vi "TemplateDaemonTester.vi"() -> ()   [LabVIEW 2024]
uses:
  TemplateDaemon_class/status--cluster.ctl
  TemplateDaemon_class/states--enum.ctl
  TemplateDaemon_class/TemplateDaemon.lvclass
  <vilib>/addons/_JKI Toolkits/State Machine/_JKI_lib_State_Machine.llb/Select State(s)_err__jki_lib_state_machine.vi
panel:
  in  "loop period (ms)":i32
  in  "set period":bool
  out "current status":T1
  in  "stop daemon":bool
  in  "start daemon":bool
  in  "destroy daemon":bool
  in  "create daemon":bool
  in  "Exit":bool
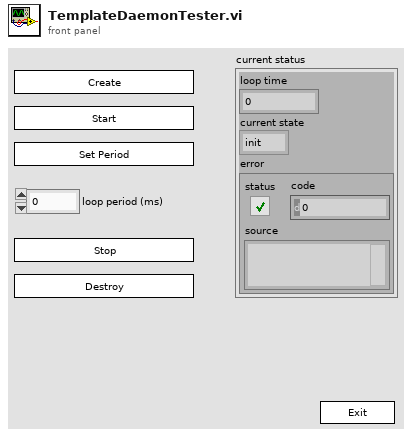
[diagram p1: front panel]
types:
  T1 = typedef "TemplateDaemon.lvclass/status--cluster.ctl" = cluster{"loop time":u32, "current state":T2, "error":errorcluster}
  T2 = typedef "TemplateDaemon.lvclass/states--enum.ctl" = enum16{"init", "default", "error handler", "exit"}
  T3 = enum32{"Invalid", "Standard", "Closed", "Hidden", "Minimized", "Maximized"}
  T4 = enum32{"invalid app kind", "Development System", "Run Time System", "Student Edition", "Embedded LabVIEW", "Evaluation", "Custom"}
  T5 = cluster{"Core":cluster{"Current VI Reference":refnum<vi>, "Close Panel on Exit?":bool}, "TemplateDaemon":refnum<class "TemplateDaemon.lvclass">, "TO":i32}
  T6 = cluster{"Current VI Reference":refnum<vi>, "Close Panel on Exit?":bool}
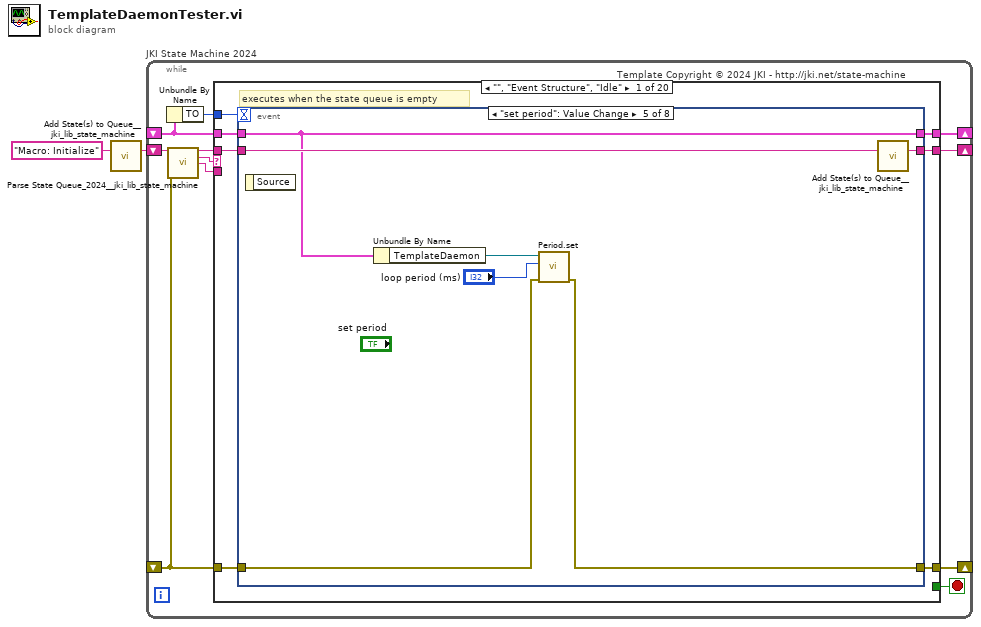
[diagram p0: block diagram]
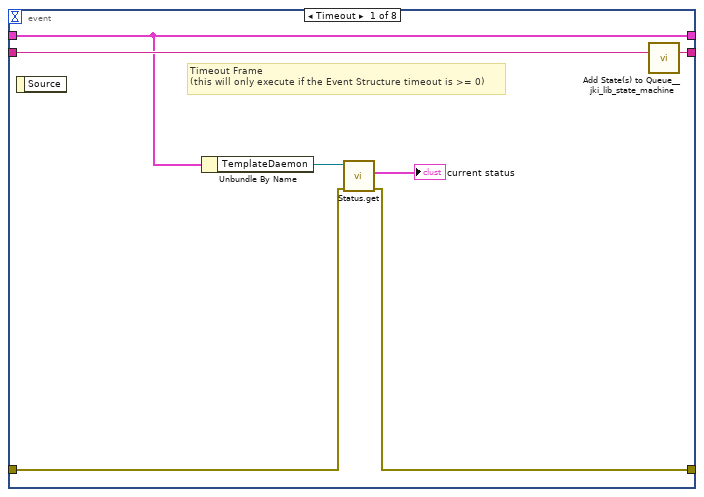
[diagram p2: hidden frame]
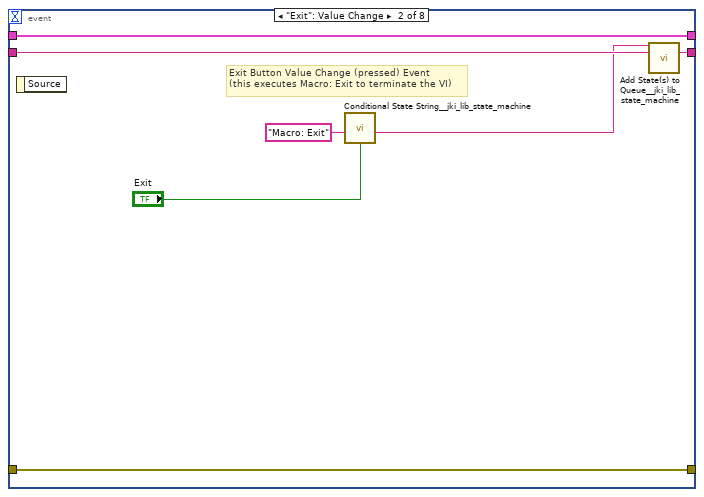
[diagram p3: hidden frame]
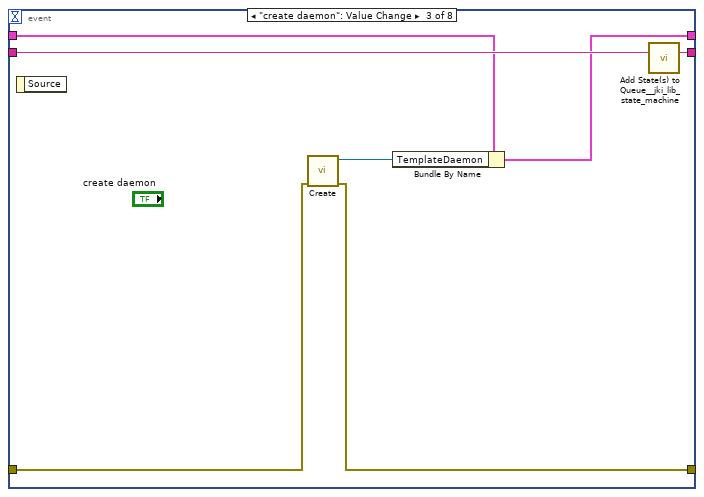
[diagram p4: hidden frame]
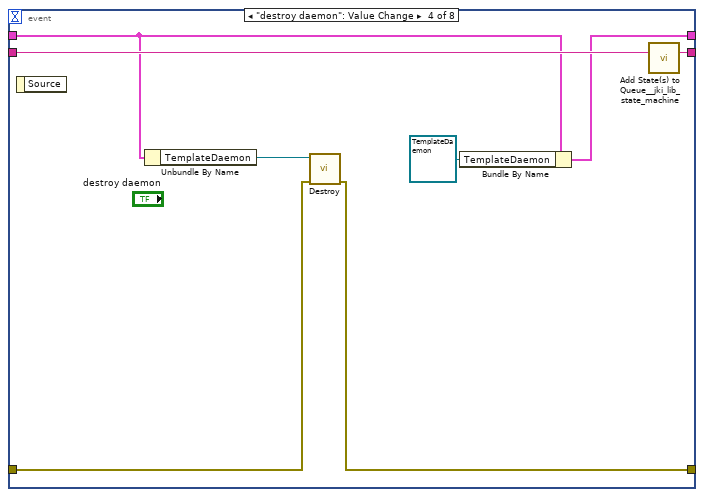
[diagram p5: hidden frame]
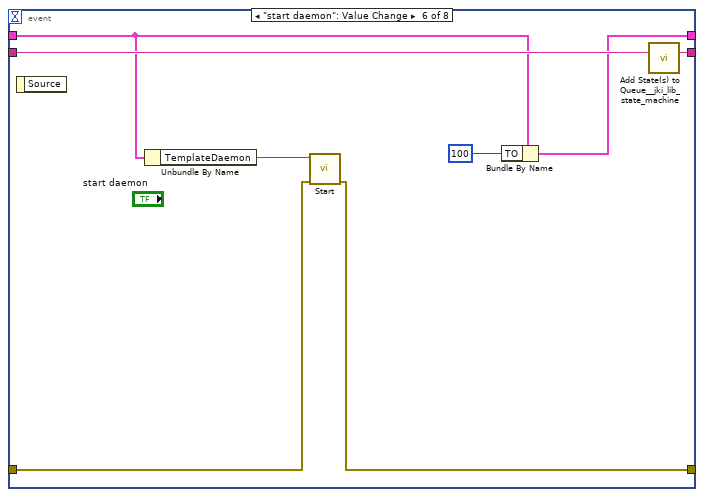
[diagram p6: hidden frame]
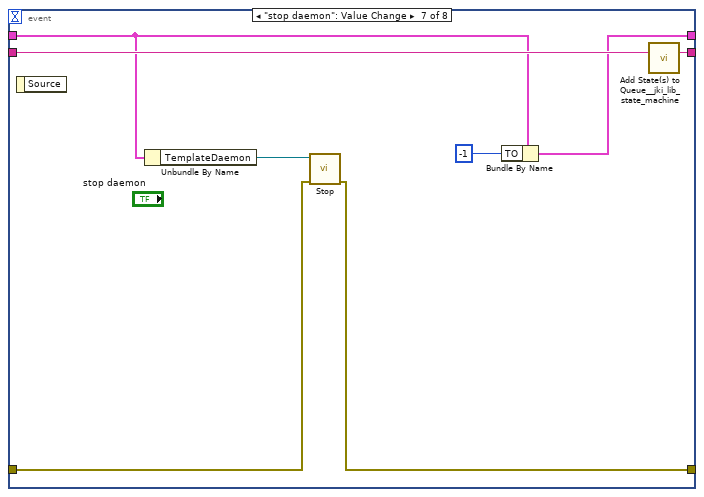
[diagram p7: hidden frame]
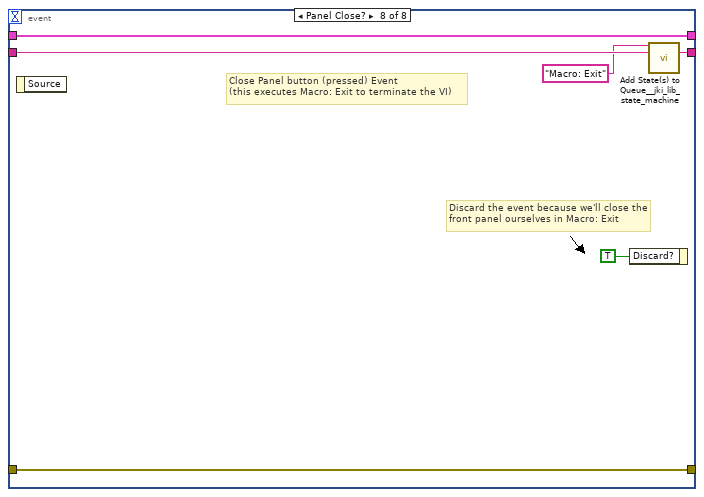
[diagram p8: hidden frame]
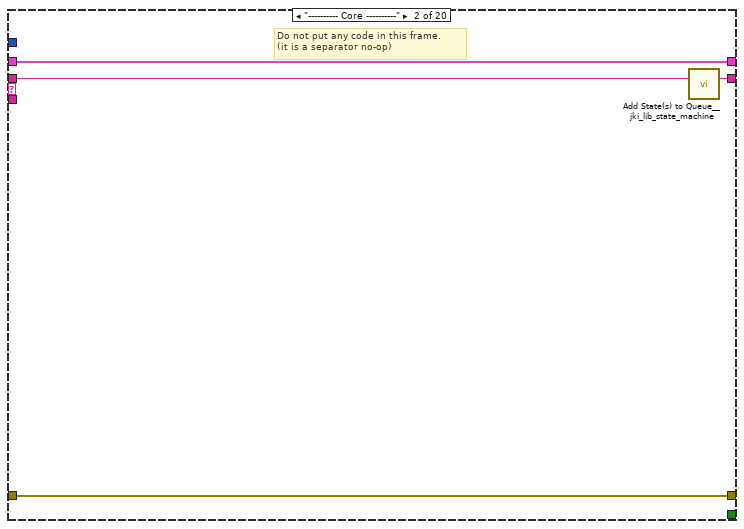
[diagram p9: hidden frame]
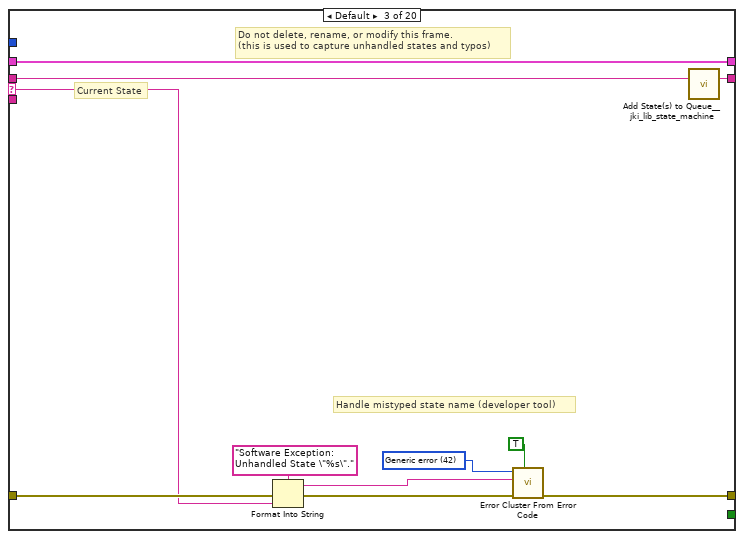
[diagram p10: hidden frame]
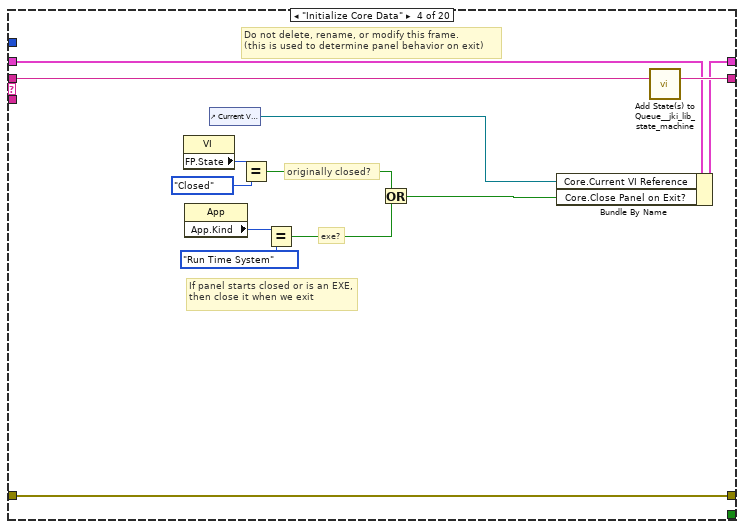
[diagram p11: hidden frame]
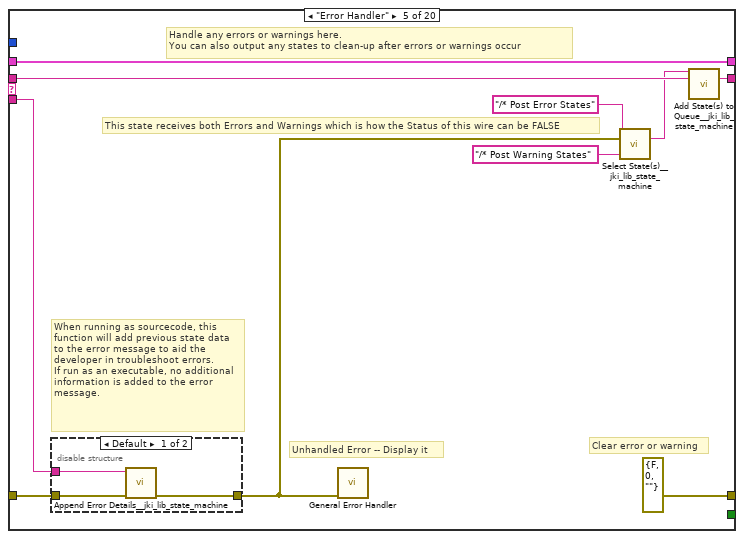
[diagram p12: hidden frame]
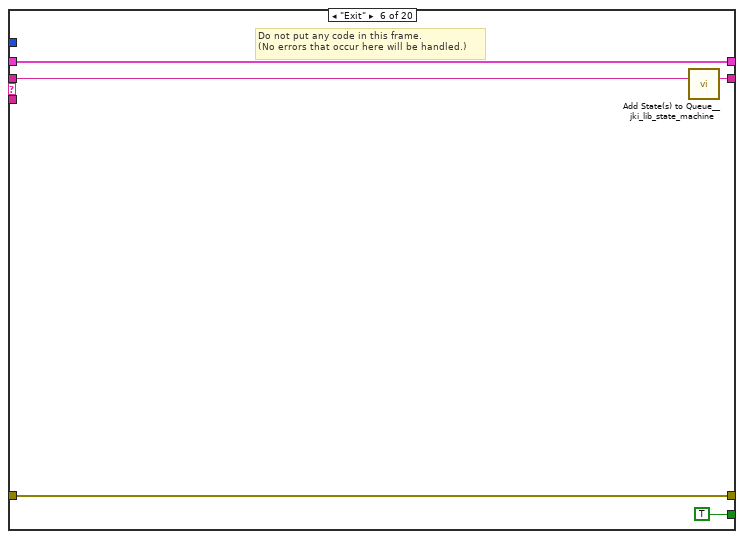
[diagram p14: hidden frame]
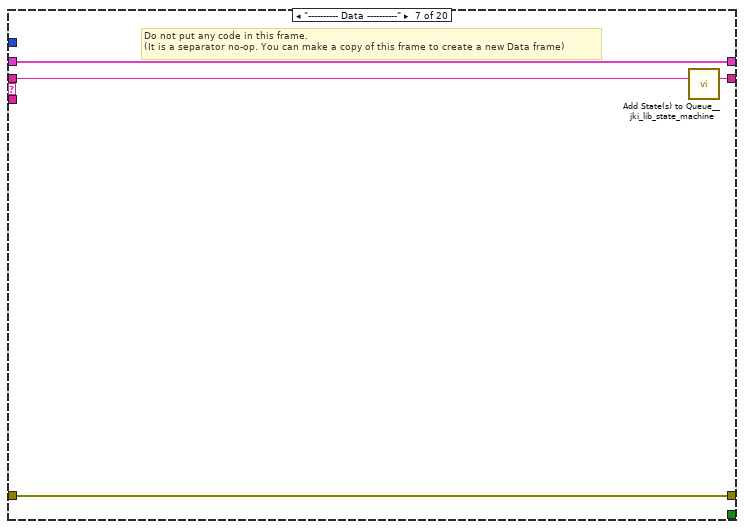
[diagram p15: hidden frame]
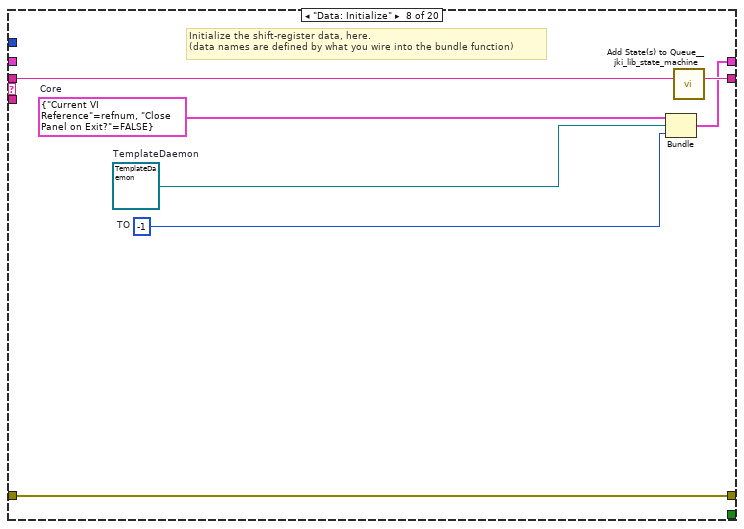
[diagram p16: hidden frame]
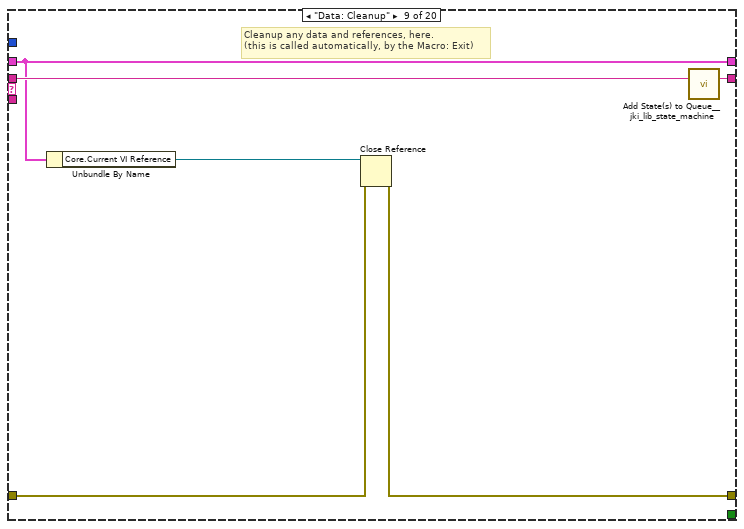
[diagram p17: hidden frame]
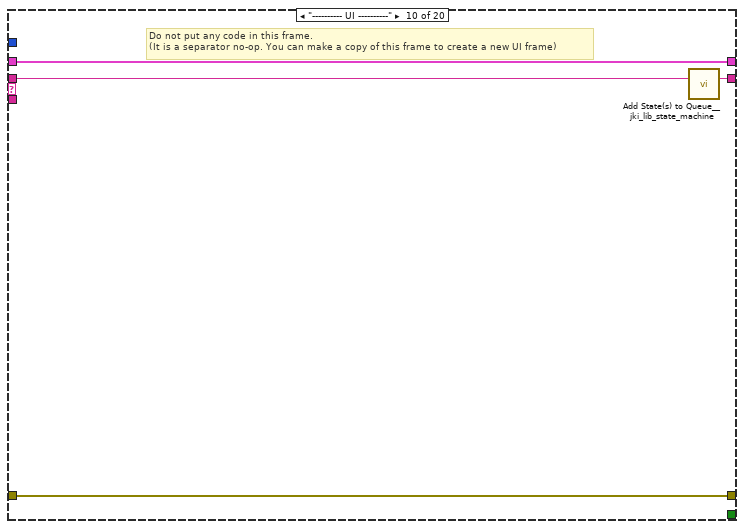
[diagram p18: hidden frame]
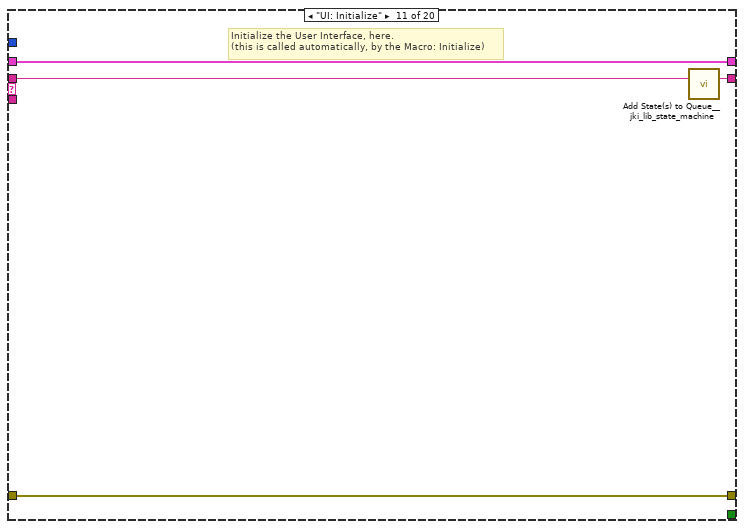
[diagram p19: hidden frame]
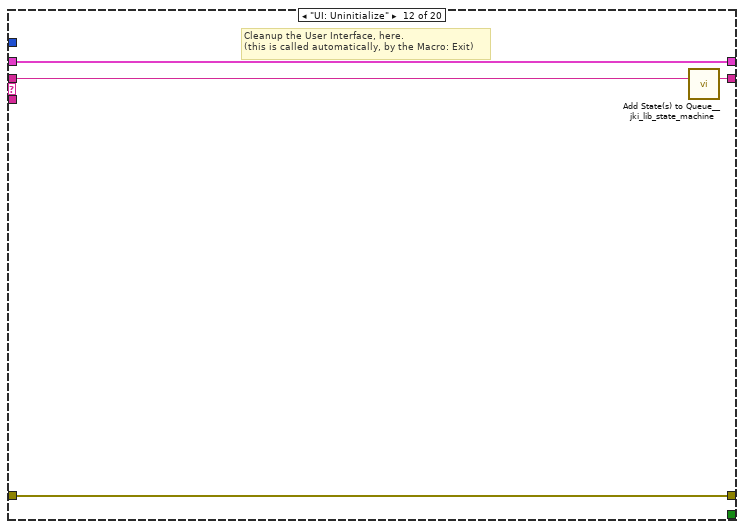
[diagram p20: hidden frame]
diagram:
  n1 = call <vilib>:"Add State(s) to Queue__jki_lib_state_machine.vi"("State(s) in (\"\")"="Macro: Initialize") -> ("States Out"=w2:string)  [unwired: 14 in]
  n2 = while "JKI State Machine 2024" {
    shift-right: [w6] -> _
    shift-left: _ -> [w4]
    shift-right: [w9] -> _
    shift-left: _ -> [w5]
    shift-right: [w8] -> _
    shift-left: w2 -> [w10]
    stop <- w7 stop-if-true
    # "Template Copyright © 2024 JKI - http://jki.net/state-machine"
    n3 = Unbundle By Name(w4) -> ("TO"=w3:i32)
    n4 = call <vilib>:"Parse State Queue_2024__jki_lib_state_machine.vi"("State Queue"=w10, "Error In (no error)"=w5) -> ("Remaining States"=w12:string, "Current State"=w13:string, "Arguments"=w11:string)  [unwired: 11 in]
    n5 = case shown="\"\", \"Event Structure\", \"Idle\"" w13 {
      selector: w13 -> [_ _ w83 _ _ _ _ _ _ _ _ _ _ _ _ _ _ _ _ _]
      tunnel: w12 -> [w20 w82 w87 w106 w116 w125 w129 w136 w142 w146 w150 w154 w160 w171 w240 w245 w254 w258 w262 w266]
      tunnel: w11 -> [_ _ _ _ w111 _ _ _ _ _ _ _ w155 w165 _ _ _ _ _ _]
      tunnel: w4 -> [w18 w79 w85 w99 w113 w123 w126 _ w137 w143 w148 w152 w158 w167 w237 w242 w252 w255 w259 w263]
      tunnel: [w17 w80 w89 w103 errorcluster {"status"=FALSE, "code"=0, "source"=""} ("error out") w122 w127 w133 w138 w144 w147 w151 w156 w168 w238 w243 w249 w256 w260 w264] -> w9
      tunnel: w5 -> [w14 w80 w88 w103 w112 w122 w127 w133 w139 w144 w147 w151 w157 w169 w238 w243 w249 w256 w260 w264]
      tunnel: [w19 w81 w86 w105 w115 w124 w128 w135 w141 w145 w149 w153 w159 w170 w239 w244 w253 w257 w261 w265] -> w8
      tunnel: [_ _ _ _ _ TRUE _ _ _ _ _ _ _ _ _ _ _ _ _ _] -> w7
      tunnel: [w16 w79 w85 w104 w113 w123 w126 w134 w137 w143 w148 w152 w158 w167 w237 w242 w252 w255 w259 w263] -> w6
      tunnel: w3 -> [w15 _ _ _ _ _ _ _ _ _ _ _ _ _ _ _ _ _ _ _]
      frame "", "Event Structure", "Idle" {
        # "executes when the state queue is empty"
        n6 = event shown="[4] \"set period\": Value Change" {
          selector: _ -> [_ _ _ _ _ _ _ _]
          dyn-events: _ -> [_ _ _ _ _ _ _ _]
          timeout: w15 -> [_ _ _ _ _ _ _ _]
          tunnel: w20 -> [w27 w34 w41 w49 w56 w64 w72 w78]
          tunnel: [w26 w33 w40 w48 w55 w63 w71 w77] -> w19
          tunnel: w18 -> [w25 w31 w39 w43 w52 w59 w67 w75]
          tunnel: [w22 w32 w35 w45 w53 w61 w69 w76] -> w17
          tunnel: w14 -> [w23 w32 w36 w46 w54 w62 w70 w76]
          tunnel: [w25 w31 w38 w47 w52 w58 w66 w75] -> w16
          event Timeout {
            # "Timeout Frame\n(this will only execute if the Event Structure timeout is >= 0)"
            n7 = event-data() -> ()  [unwired: 1 in, 1 out]
            n8 = Unbundle By Name(w25) -> ("TemplateDaemon"=w24:refnum<class "TemplateDaemon.lvclass">)
            n9 = call "Status.get.vi"("error in (no error)"=w23, "EventDaemon in"=w24) -> ("error out"=w22:errorcluster, "current status"=→"current status":T1)  [unwired: 7 in, 1 out]
            n10 = call <vilib>:"Add State(s) to Queue__jki_lib_state_machine.vi"("State(s) in (\"\")"=w27) -> ("States Out"=w26:string)  [unwired: 14 in]
          }
          event "Exit": Value Change {
            # "Exit Button Value Change (pressed) Event\n(this executes Macro: Exit to terminate the VI)"
            n11 = event-data() -> ()  [unwired: 1 in, 1 out]
            n12 = call <vilib>:"Conditional State String__jki_lib_state_machine.vi"("Do State(s)?"="Exit", "State"="Macro: Exit") -> ("State Out"=w28:string)  [unwired: 7 in]
            n13 = call <vilib>:"Add State(s) to Queue__jki_lib_state_machine.vi"("State(s) in Front (\"\")"=w28, "State(s) in (\"\")"=w34) -> ("States Out"=w33:string)  [unwired: 13 in]
          }
          event "create daemon": Value Change {
            n14 = event-data() -> ()  [unwired: 1 in, 1 out]
            n15 = call "Create.vi"("error in (no error)"=w36) -> ("error out"=w35:errorcluster, "EventDaemon out"=w37:refnum<class "TemplateDaemon.lvclass">)  [unwired: 9 in]
            n16 = Bundle By Name(cluster=w39, "TemplateDaemon"=w37) -> (w38:T5)
            n17 = call <vilib>:"Add State(s) to Queue__jki_lib_state_machine.vi"("State(s) in (\"\")"=w41) -> ("States Out"=w40:string)  [unwired: 14 in]
          }
          event "destroy daemon": Value Change {
            n18 = event-data() -> ()  [unwired: 1 in, 1 out]
            n19 = Unbundle By Name(w43) -> ("TemplateDaemon"=w42:refnum<class "TemplateDaemon.lvclass">)
            n20 = call-dynamic "Destroy.vi"("error in (no error)"=w46, "EventDaemon in"=w42) -> ("error out"=w45:errorcluster)  [unwired: 9 in]
            n21 = Bundle By Name(cluster=w43, "TemplateDaemon"=refnum<class "TemplateDaemon.lvclass"> refnum) -> (w47:T5)
            n22 = call <vilib>:"Add State(s) to Queue__jki_lib_state_machine.vi"("State(s) in (\"\")"=w49) -> ("States Out"=w48:string)  [unwired: 14 in]
          }
          event "set period": Value Change {
            n23 = event-data() -> ()  [unwired: 1 in, 1 out]
            n24 = Unbundle By Name(w52) -> ("TemplateDaemon"=w51:refnum<class "TemplateDaemon.lvclass">)
            n25 = call "Period.set.vi"("error in (no error)"=w54, "period (ms)"="loop period (ms)", "EventDaemon in"=w51) -> ("error out"=w53:errorcluster)  [unwired: 7 in, 1 out]
            n26 = call <vilib>:"Add State(s) to Queue__jki_lib_state_machine.vi"("State(s) in (\"\")"=w56) -> ("States Out"=w55:string)  [unwired: 14 in]
          }
          event "start daemon": Value Change {
            n27 = event-data() -> ()  [unwired: 1 in, 1 out]
            n28 = Unbundle By Name(w59) -> ("TemplateDaemon"=w60:refnum<class "TemplateDaemon.lvclass">)
            n29 = call-dynamic "Start.vi"("error in (no error)"=w62, "EventDaemon in"=w60) -> ("error out"=w61:errorcluster)  [unwired: 8 in, 1 out]
            n30 = Bundle By Name(cluster=w59, "TO"=100) -> (w58:T5)
            n31 = call <vilib>:"Add State(s) to Queue__jki_lib_state_machine.vi"("State(s) in (\"\")"=w64) -> ("States Out"=w63:string)  [unwired: 14 in]
          }
          event "stop daemon": Value Change {
            n32 = event-data() -> ()  [unwired: 1 in, 1 out]
            n33 = Unbundle By Name(w67) -> ("TemplateDaemon"=w68:refnum<class "TemplateDaemon.lvclass">)
            n34 = call "Stop.vi"("error in (no error)"=w70, "EventDaemon in"=w68) -> ("error out"=w69:errorcluster)  [unwired: 8 in, 1 out]
            n35 = Bundle By Name(cluster=w67, "TO"=-1) -> (w66:T5)
            n36 = call <vilib>:"Add State(s) to Queue__jki_lib_state_machine.vi"("State(s) in (\"\")"=w72) -> ("States Out"=w71:string)  [unwired: 14 in]
          }
          event Panel Close? {
            # "Discard the event because we'll close the front panel ourselves in Macro: Exit"
            # "Close Panel button (pressed) Event\n(this executes Macro: Exit to terminate the VI)"
            n37 = event-data() -> ()  [unwired: 1 in, 1 out]
            n38 = event-data("Discard?"=TRUE) -> ()  [unwired: 1 in, 1 out]
            n39 = call <vilib>:"Add State(s) to Queue__jki_lib_state_machine.vi"("State(s) in Front (\"\")"="Macro: Exit", "State(s) in (\"\")"=w78) -> ("States Out"=w77:string)  [unwired: 13 in]
          }
        }
      }
      frame "---------- Core ----------" {
        # "Do not put any code in this frame.\n(it is a separator no-op)"
        n40 = call <vilib>:"Add State(s) to Queue__jki_lib_state_machine.vi"("State(s) in (\"\")"=w82) -> ("States Out"=w81:string)  [unwired: 14 in]
      }
      frame Default {
        w92 = 42 items=["No error", "Argument error", "Memory is full", "Out of zone", "End of file", "File already open", "Generic file I/O error", "File not found", "File permission error", "Disk is full", "Duplicate path", "Too many files open", "System feature not enabled", "Resource file not found", "Cannot add resource", "Resource not found", "Image not found", "Image memory error", "Pen does not exist", "Config type invalid", "Config token not found", "Config parse error", "Config memory error", "Bad external code format", "Bad external code offset", "External code not present", "Null window", "Destroy window error", "Null menu", "Print aborted", "Bad print record", "Print driver error", "Windows error during printing", "Memory error during printing", "Print dialog error", "Generic print error", "Invalid device refnum", "Device not found", "Device parameter error", "Device unit error", "Cannot open device", "Device call aborted", "Generic error", "Cancelled by user", "Object ID too low", "Object ID too high", "Object not in heap", "Unknown heap", "Unknown object (invalid DefProc)", "Unknown object (DefProc not in table)", "Message out of range", "Invalid (null) method", "Unknown message", "Manager call not supported", "Bad address", "Network operation in progress", "Network operation timed out", "Connection is busy", "Network attribute not supported", "Network error", "Address in use", "System out of memory", "Connection aborted", "Connection refused", "Not connected", "Already connected", "Connection closed", "Initialization error (interapplication manager)", "Bad occurrence", "Wait on unbound occurrence handler", "Occurrence queue overflow", "Datalog type conflict", "Unused", "Unrecognized type (interapplication manager)", "Memory corrupt", "Failed to make temporary DLL", "Old CIN version", "Drag socket not found", "Failed to load drop-object", "Failed to register OLE object", "Failed to release OLE object", "Format specifier type mismatch", "Unknown format specifier", "Too few format specifiers", "Too many format specifiers", "Scan failed", "Newer CIN version", "Error converting to variant", "Runtime menu error", "Password tampered", "Variant attribute not found", "Incompatible variant data type", "Event data is not available", "Event Store is not present", "Occurrence is not found", "Event Queue is not created", "Event info is not available", "Refnum passed is NULL", "Error retrieving Class GUID", "Error retrieving CoClass GUID", "Error retrieving TypeLib GUID.", "Bad built application magic bytes.", "Specific driver is different from the specific driver associated with the Logical Name.", "There is no session opened to the class driver.", "Max Error", "MAX - Error with config objects", "MAX - Error loading configuration", "MAX - Group not supported"]
        # "Current State"
        # "Do not delete, rename, or modify this frame.\n(this is used to capture unhandled states and typos)"
        # "Handle mistyped state name (developer tool)"
        n41 = Format Into String(format string="Software Exception: Unhandled State \"%s\"." ("message"), error in=w88, w83) -> (resulting string=w91:string, error out=w90:errorcluster)  [unwired: 1 in]
        n42 = call <vilib>:"Error Cluster From Error Code.vi"("show call chain? (False)"=TRUE, "error in (no error)"=w90, "error message (\"\")"=w91, "error code (0)"=w92) -> ("error out"=w89:errorcluster)  [unwired: 5 in]
        n43 = call <vilib>:"Add State(s) to Queue__jki_lib_state_machine.vi"("State(s) in (\"\")"=w87) -> ("States Out"=w86:string)  [unwired: 14 in]
      }
      frame "Initialize Core Data" {
        # "Do not delete, rename, or modify this frame.\n(this is used to determine panel behavior on exit)"
        # "originally closed?"
        # "exe?"
        # "If panel starts closed or is an EXE, then close it when we exit"
        n44 = property class="VI"() -> ("FP.State"=w96:T3)  [unwired: 2 in, 2 out]
        n45 = property class="App"() -> ("App.Kind"=w102:T4)  [unwired: 2 in, 2 out]
        n46 = control-ref of="Current VI Reference"() -> (w97:refnum<vi>)
        n47 = Equal?(x=w96, y=T3."Closed" ("Front Panel Window:State")) -> (x = y?=w94:bool)
        n48 = Equal?(x=w102, y=T4."Run Time System" ("Application:Kind")) -> (x = y?=w100:bool)
        n49 = Or(x=w94, y=w100) -> (x .or. y?=w98:bool)
        n50 = Bundle By Name(cluster=w99, "Core.Current VI Reference"=w97, "Core.Close Panel on Exit?"=w98) -> (w104:T5)
        n51 = call <vilib>:"Add State(s) to Queue__jki_lib_state_machine.vi"("State(s) in (\"\")"=w106) -> ("States Out"=w105:string)  [unwired: 14 in]
      }
      frame "Error Handler" {
        # "When running as sourcecode, this function will add previous state data to the error message to aid the developer in troubleshoot errors.\nIf run as an executable, no additional information is added to the error message."
        # "This state receives both Errors and Warnings which is how the Status of this wire can be FALSE"
        # "Unhandled Error -- Display it"
        # "Handle any errors or warnings here.\nYou can also output any states to clean-up after errors or warnings occur"
        # "Clear error or warning"
        n52 = disable-structure shown="Default" {
          disable-tunnel: w112 -> [w119 w120]
          disable-tunnel: w111 -> [w118 _]
          disable-tunnel: [w117 w120] -> w110
          frame condition #0 (active) {
            n53 = call <vilib>:"Append Error Details__jki_lib_state_machine.vi"("error in (no error)"=w119, "Previous State and Argument(s)"=w118) -> ("error out"=w117:errorcluster)  [unwired: 9 in]
          }
          frame condition #1 {
          }
        }
        n54 = call <vilib>:"General Error Handler.vi"("error in (no error)"=w110) -> ()  [unwired: 10 in, 5 out]
        n55 = call-poly <vilib>:"Select State(s)__jki_lib_state_machine.vi"("State(s) if True (\"\")"="/* Post Error States", "Select"=w110, "State(s) if False (\"\")"="/* Post Warning States") -> ("States Out"=w108:string)  [unwired: 12 in]
        n56 = call <vilib>:"Add State(s) to Queue__jki_lib_state_machine.vi"("State(s) in Front (\"\")"=w108, "State(s) in (\"\")"=w116) -> ("States Out"=w115:string)  [unwired: 13 in]
      }
      frame "Exit" {
        # "Do not put any code in this frame.\n(No errors that occur here will be handled.)"
        n57 = call <vilib>:"Add State(s) to Queue__jki_lib_state_machine.vi"("State(s) in (\"\")"=w125) -> ("States Out"=w124:string)  [unwired: 14 in]
      }
      frame "---------- Data ----------" {
        # "Do not put any code in this frame.\n(It is a separator no-op. You can make a copy of this frame to create a new Data frame)"
        n58 = call <vilib>:"Add State(s) to Queue__jki_lib_state_machine.vi"("State(s) in (\"\")"=w129) -> ("States Out"=w128:string)  [unwired: 14 in]
      }
      frame "Data: Initialize" {
        w130 = -1  # TO
        w131 = refnum<class "TemplateDaemon.lvclass"> refnum  # TemplateDaemon
        w132 = T6 {"Current VI Reference"=refnum, "Close Panel on Exit?"=FALSE}  # Core
        # "Initialize the shift-register data, here.\n(data names are defined by what you wire into the bundle function)"
        n59 = Bundle("Core"=w132, "TemplateDaemon"=w131, "TO"=w130) -> (w134:T5)  [unwired: 1 in]
        n60 = call <vilib>:"Add State(s) to Queue__jki_lib_state_machine.vi"("State(s) in (\"\")"=w136) -> ("States Out"=w135:string)  [unwired: 14 in]
      }
      frame "Data: Cleanup" {
        # "Cleanup any data and references, here.\n(this is called automatically, by the Macro: Exit)"
        n61 = Unbundle By Name(w137) -> ("Core.Current VI Reference"=w140:refnum<vi>)
        n62 = Close Reference(reference=w140, error in (no error)=w139) -> (error out=w138:errorcluster)
        n63 = call <vilib>:"Add State(s) to Queue__jki_lib_state_machine.vi"("State(s) in (\"\")"=w142) -> ("States Out"=w141:string)  [unwired: 14 in]
      }
      frame "---------- UI ----------" {
        # "Do not put any code in this frame.\n(It is a separator no-op. You can make a copy of this frame to create a new UI frame)"
        n64 = call <vilib>:"Add State(s) to Queue__jki_lib_state_machine.vi"("State(s) in (\"\")"=w146) -> ("States Out"=w145:string)  [unwired: 14 in]
      }
      frame "UI: Initialize" {
        # "Initialize the User Interface, here.\n(this is called automatically, by the Macro: Initialize)"
        n65 = call <vilib>:"Add State(s) to Queue__jki_lib_state_machine.vi"("State(s) in (\"\")"=w150) -> ("States Out"=w149:string)  [unwired: 14 in]
      }
      frame "UI: Uninitialize" {
        # "Cleanup the User Interface, here.\n(this is called automatically, by the Macro: Exit)"
        n66 = call <vilib>:"Add State(s) to Queue__jki_lib_state_machine.vi"("State(s) in (\"\")"=w154) -> ("States Out"=w153:string)  [unwired: 14 in]
      }
      frame "UI: Cursor Set" {
        # "Argument"
        # "Set and Unset Cursor Busy.\n(Usage: \"UI: Cursor Set >> Busy|Idle\")"
        n67 = case shown="\"Idle\", Default" w155 {
          tunnel: w157 -> [w162 w164]
          tunnel: [w161 w163] -> w156
          frame "Idle", Default {
            n68 = call <vilib>:"Unset Busy.vi"("error in (no error)"=w162) -> ("error out"=w161:errorcluster)  [unwired: 10 in]
          }
          frame "Busy" {
            n69 = call <vilib>:"Set Busy.vi"("error in (no error)"=w164) -> ("error out"=w163:errorcluster)  [unwired: 9 in, 1 out]
          }
        }
        n70 = call <vilib>:"Add State(s) to Queue__jki_lib_state_machine.vi"("State(s) in (\"\")"=w160) -> ("States Out"=w159:string)  [unwired: 14 in]
      }
      frame "UI: Front Panel State" {
        # "Argument"
        # "Set Front Panel Open or Closed\n(Usage: \"UI: Front Panel State >> Open|Close\")"
        n71 = Unbundle By Name(w167) -> ("Core.Current VI Reference"=w166:refnum<vi>)
        n72 = case shown="\"Minimize\", \"Minimized\"" w165 {
          tunnel: w169 -> [w177 w192 w203 w216 w229]
          tunnel: [w179 w193 w205 w218 w231] -> w168
          tunnel: w166 -> [w178 w190 w204 w217 w230]
          frame "Open", "Standard", Default {
            w172 = T3."Standard" ("State")
            n73 = property class="VI"(reference=w178, error in=w177) -> (reference out=w175:refnum<vi>, error out=w176:errorcluster, "FP.State"=w174:T3)
            n74 = Not Equal?(x=w174, y=w172) -> (x != y?=w173:bool)
            n75 = case shown="True" w173 {
              tunnel: [w183 w185] -> w179
              tunnel: w176 -> [w182 w185]
              tunnel: w175 -> [w181 _]
              tunnel: w172 -> [w180 _]
              frame True {
                n76 = invoke class="VI" method="FP.Open"(reference=w181, error in=w182, "Activate"=TRUE, "State"=w180) -> (error out=w183:errorcluster)  [unwired: 1 in, 4 out]
              }
              frame False {
              }
            }
          }
          frame "Close", "Closed" {
            n77 = property class="VI"(reference=w190, error in=w192) -> (reference out=w189:refnum<vi>, error out=w191:errorcluster, "FP.State"=w187:T3)
            n78 = Not Equal?(x=w187, y=T3."Closed" ("Front Panel Window:State")) -> (x != y?=w186:bool)
            n79 = case shown="True" w186 {
              tunnel: [w194 w197] -> w193
              tunnel: w191 -> [w194 w196]
              tunnel: w189 -> [_ w195]
              frame False {
              }
              frame True {
                n80 = invoke class="VI" method="FP.Close"(reference=w195, error in=w196) -> (error out=w197:errorcluster)  [unwired: 1 in, 2 out]
              }
            }
          }
          frame "Hidden", "Hide" {
            w198 = T3."Hidden" ("State")
            n81 = property class="VI"(reference=w204, error in=w203) -> (reference out=w201:refnum<vi>, error out=w202:errorcluster, "FP.State"=w200:T3)
            n82 = Not Equal?(x=w200, y=w198) -> (x != y?=w199:bool)
            n83 = case shown="True" w199 {
              tunnel: [w209 w210] -> w205
              tunnel: w202 -> [w208 w210]
              tunnel: w201 -> [w207 _]
              tunnel: w198 -> [w206 _]
              frame True {
                n84 = invoke class="VI" method="FP.Open"(reference=w207, error in=w208, "State"=w206) -> (error out=w209:errorcluster)  [unwired: 2 in, 4 out]
              }
              frame False {
              }
            }
          }
          frame "Minimize", "Minimized" {
            w211 = T3."Minimized" ("State")
            n85 = property class="VI"(reference=w217, error in=w216) -> (reference out=w214:refnum<vi>, error out=w215:errorcluster, "FP.State"=w213:T3)
            n86 = Not Equal?(x=w213, y=w211) -> (x != y?=w212:bool)
            n87 = case shown="True" w212 {
              tunnel: [w222 w223] -> w218
              tunnel: w215 -> [w221 w223]
              tunnel: w214 -> [w220 _]
              tunnel: w211 -> [w219 _]
              frame True {
                n88 = invoke class="VI" method="FP.Open"(reference=w220, error in=w221, "State"=w219) -> (error out=w222:errorcluster)  [unwired: 2 in, 4 out]
              }
              frame False {
              }
            }
          }
          frame "Maximize", "Maximized" {
            w224 = T3."Maximized" ("State")
            n89 = property class="VI"(reference=w230, error in=w229) -> (reference out=w227:refnum<vi>, error out=w228:errorcluster, "FP.State"=w226:T3)
            n90 = Not Equal?(x=w226, y=w224) -> (x != y?=w225:bool)
            n91 = case shown="True" w225 {
              tunnel: [w235 w236] -> w231
              tunnel: w228 -> [w234 w236]
              tunnel: w227 -> [w233 _]
              tunnel: w224 -> [w232 _]
              frame True {
                n92 = invoke class="VI" method="FP.Open"(reference=w233, error in=w234, "State"=w232) -> (error out=w235:errorcluster)  [unwired: 2 in, 4 out]
              }
              frame False {
              }
            }
          }
        }
        n93 = call <vilib>:"Add State(s) to Queue__jki_lib_state_machine.vi"("State(s) in (\"\")"=w171) -> ("States Out"=w170:string)  [unwired: 14 in]
      }
      frame "---------- Macro ----------" {
        # "Do not put any code in this frame.\n(It is a separator no-op. You can make a copy of this frame to create a new Macro frame)"
        n94 = call <vilib>:"Add State(s) to Queue__jki_lib_state_machine.vi"("State(s) in (\"\")"=w240) -> ("States Out"=w239:string)  [unwired: 14 in]
      }
      frame "Macro: Initialize" {
        w241 = "Data: Initialize\nInitialize Core Data\nUI: Initialize\nUI: Front Panel State >> Open"  # Data: Initialize Initialize Core Data UI: Initialize UI: Front Panel State >> Open
        # "Initialization Macro\n(This is called once, when the VI starts)"
        n95 = call <vilib>:"Add State(s) to Queue__jki_lib_state_machine.vi"("State(s) in Front (\"\")"=w241, "State(s) in (\"\")"=w245) -> ("States Out"=w244:string)  [unwired: 13 in]
      }
      frame "Macro: Exit" {
        # "Exit Macro\n(This is called once, when the VI exits)"
        n96 = Unbundle By Name(w252) -> ("Core.Close Panel on Exit?"=w247:bool)
        n97 = call <vilib>:"Conditional State String__jki_lib_state_machine.vi"("Do State(s)?"=w247, "State"="UI: Front Panel State >> Close") -> ("State Out"=w246:string)  [unwired: 7 in]
        n98 = call <vilib>:"Add State(s) to Queue__jki_lib_state_machine.vi"("State(s) in (\"\")"=w246, "State(s) at Back (\"\")"="UI: Uninitialize\nData: Cleanup\nExit") -> ("States Out"=w250:string)  [unwired: 13 in]
        n99 = call <vilib>:"Add State(s) to Queue__jki_lib_state_machine.vi"("State(s) in Front (\"\")"=w250, "State(s) in (\"\")"=w254) -> ("States Out"=w253:string)  [unwired: 13 in]
      }
      frame "---------- New Category ----------" {
        # "Template Separator\n(You can make a copy of, or modify, this frame)"
        n100 = call <vilib>:"Add State(s) to Queue__jki_lib_state_machine.vi"("State(s) in (\"\")"=w258) -> ("States Out"=w257:string)  [unwired: 14 in]
      }
      frame "New Category: 1" {
        # "Your code here.\n(You can make a copy of, or modify, this frame)"
        n101 = call <vilib>:"Add State(s) to Queue__jki_lib_state_machine.vi"("State(s) in (\"\")"=w262) -> ("States Out"=w261:string)  [unwired: 14 in]
      }
      frame "New Category: 2" {
        # "Your code here.\n(You can make a copy of, or modify, this frame)"
        n102 = call <vilib>:"Add State(s) to Queue__jki_lib_state_machine.vi"("State(s) in (\"\")"=w266) -> ("States Out"=w265:string)  [unwired: 14 in]
      }
    }
  }
